vi "HexToCDABFloat.vi"(11 "数组":u16[](array[numeric]) format="%04xH") -> (3 "FLOAT":sgl[](array[numeric]))   [LabVIEW 2016, in "质控单元.lvlib"]
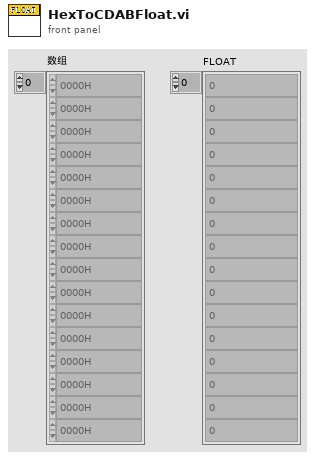
[diagram p1: front panel]
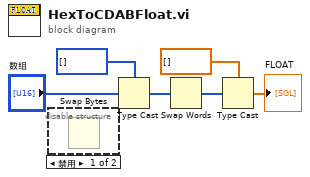
[diagram p0: block diagram]
diagram:
  n1 = disable-structure shown="禁用" {
    frame Disabled {
      n2 = Swap Bytes() -> ()  [unwired: 1 in, 1 out]
    }
    frame Enabled {
    }
  }
  n3 = Type Cast(type=u32[] [], x="数组") -> (*(type *) &x=w3:u32[])
  n4 = Swap Words(1:w3) -> (0:w2:u32[])
  n5 = Type Cast(type=sgl[] [], x=w2) -> (*(type *) &x=→"FLOAT":sgl[])
